vi "Get Entry by Index.vi"(8 "error in":errorcluster, 10 "Index":i32, 11 "Object Dictionary in":refnum<class "Object Dictionary.lvclass">) -> (0 "error out":errorcluster, 2 "Entry":refnum<class "Section.lvclass">, 3 "Object Dictionary out":refnum<class "Object Dictionary.lvclass">)   [LabVIEW 2024, in "EDS.lvlib" / "Object Dictionary.lvclass"]
uses:
  Object Dictionary.lvclass
  Object Dictionary.lvclass/Object Dictionary.ctl
  OD Section/Section.lvclass
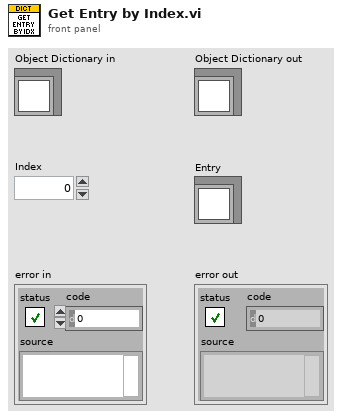
[diagram p1: front panel]
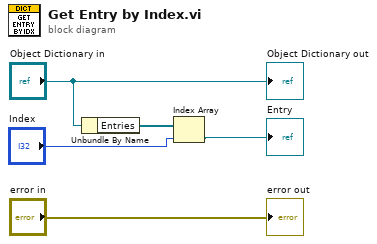
[diagram p0: block diagram]
diagram:
  n1 = Unbundle By Name("Object Dictionary in") -> ("Entries"=w3:refnum<class "Section.lvclass">[])
  n2 = Index Array(array=w3, index="Index") -> (element=→"Entry":refnum<class "Section.lvclass">)
  "error out" <- "error in"
  "Object Dictionary out" <- "Object Dictionary in"
